vi "Swerve Drive.vi"(0 "Longitudinal - Y":dbl, 2 "Lateral - X":dbl, 3 "Rotational - Z":dbl) -> (1 "Front Left Speed":dbl, 4 "Back Left Angle":dbl, 5 "Front Left Angle":dbl, 6 "Front Right Speed":dbl, 7 "Front Right Angle":dbl, 8 "Back Left Speed":dbl, 9 "Back Right Speed":dbl, 10 "Back Right Angle":dbl)   [LabVIEW 2018]
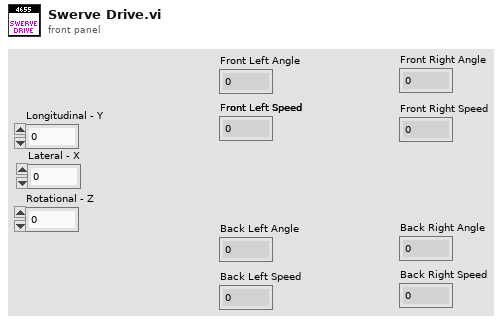
[diagram p1: front panel]
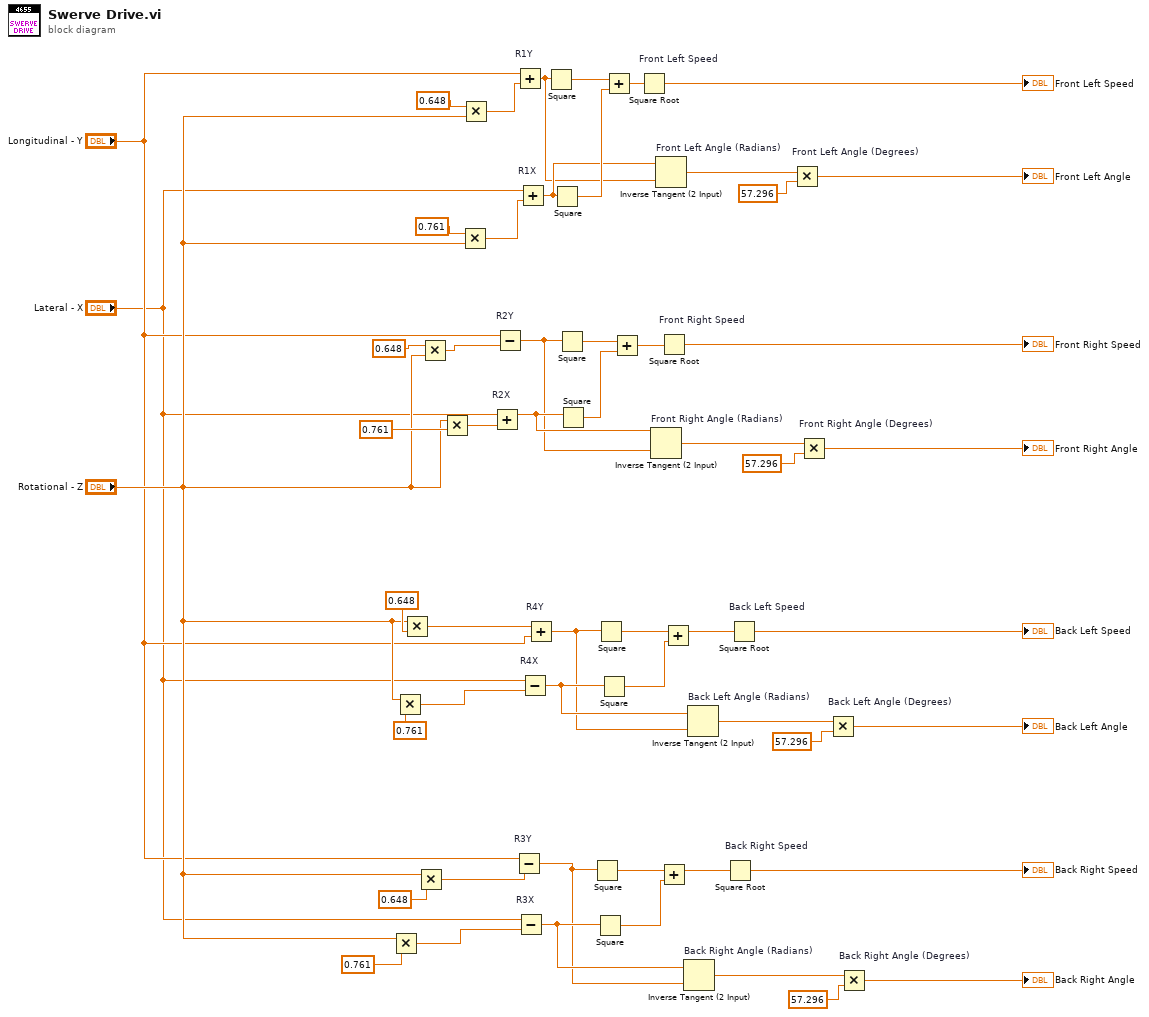
[diagram p0: block diagram]
diagram:
  n1 = Multiply(x="Rotational - Z", y=0.761 ("x")) -> (x*y=w20:dbl)
  n2 = Multiply(x="Rotational - Z", y=0.761 ("x")) -> (x*y=w30:dbl)
  n3 = Multiply(x="Rotational - Z", y=0.648 ("x")) -> (x*y=w32:dbl)
  n4 = Multiply(x="Rotational - Z", y=0.648 ("x")) -> (x*y=w11:dbl)
  n5 = Multiply(x=0.648, y="Rotational - Z") -> (x*y=w43:dbl)
  n6 = Multiply(x="Rotational - Z", y=0.761 ("x")) -> (x*y=w41:dbl)
  n7 = Multiply(x=0.761, y="Rotational - Z") -> (x*y=w52:dbl)
  n8 = Multiply(x=0.648, y="Rotational - Z") -> (x*y=w54:dbl)
  n9 = Add "R2X"(x="Lateral - X", y=w41) -> (x+y=w37:dbl)
  n10 = Subtract "R2Y"(x="Longitudinal - Y", y=w43) -> (x-y=w36:dbl)
  n11 = Subtract "R3Y"(x="Longitudinal - Y", y=w11) -> (x-y=w15:dbl)
  n12 = Add "R1Y"(x="Longitudinal - Y", y=w54) -> (x+y=w47:dbl)
  n13 = Subtract "R3X"(x="Lateral - X", y=w20) -> (x-y=w16:dbl)
  n14 = Add "R1X"(x="Lateral - X", y=w52) -> (x+y=w48:dbl)
  n15 = Subtract "R4X"(x="Lateral - X", y=w30) -> (x-y=w26:dbl)
  n16 = Add "R4Y"(x=w32, y="Longitudinal - Y") -> (x+y=w25:dbl)
  n17 = Square(x=w47) -> (x^2=w49:dbl)
  n18 = Square(x=w48) -> (x^2=w51:dbl)
  n19 = Square(x=w36) -> (x^2=w40:dbl)
  n20 = Square(x=w37) -> (x^2=w39:dbl)
  n21 = Square(x=w15) -> (x^2=w19:dbl)
  n22 = Square(x=w16) -> (x^2=w18:dbl)
  n23 = Square(x=w25) -> (x^2=w29:dbl)
  n24 = Square(x=w26) -> (x^2=w28:dbl)
  n25 = Add(x=w49, y=w51) -> (x+y=w50:dbl)
  n26 = Add(x=w40, y=w39) -> (x+y=w38:dbl)
  n27 = Square Root "Front Left Speed"(x=w50) -> (sqrt(x)=→"Front Left Speed":dbl)
  n28 = Inverse Tangent (2 Input) "Front Right Angle (Radians)"(1:w36, 2:w37) -> (0:w35:dbl)
  n29 = Inverse Tangent (2 Input) "Front Left Angle (Radians)"(1:w47, 2:w48) -> (0:w46:dbl)
  n30 = Square Root "Front Right Speed"(x=w38) -> (sqrt(x)=→"Front Right Speed":dbl)
  n31 = Add(x=w19, y=w18) -> (x+y=w17:dbl)
  n32 = Add(x=w29, y=w28) -> (x+y=w27:dbl)
  n33 = Inverse Tangent (2 Input) "Back Right Angle (Radians)"(1:w15, 2:w16) -> (0:w14:dbl)
  n34 = Inverse Tangent (2 Input) "Back Left Angle (Radians)"(1:w25, 2:w26) -> (0:w24:dbl)
  n35 = Square Root "Back Right Speed"(x=w17) -> (sqrt(x)=→"Back Right Speed":dbl)
  n36 = Square Root "Back Left Speed"(x=w27) -> (sqrt(x)=→"Back Left Speed":dbl)
  n37 = Multiply "Front Left Angle (Degrees)"(x=w46, y=57.296) -> (x*y=→"Front Left Angle":dbl)
  n38 = Multiply "Front Right Angle (Degrees)"(x=w35, y=57.296) -> (x*y=→"Front Right Angle":dbl)
  n39 = Multiply "Back Left Angle (Degrees)"(x=w24, y=57.296) -> (x*y=→"Back Left Angle":dbl)
  n40 = Multiply "Back Right Angle (Degrees)"(x=w14, y=57.296) -> (x*y=→"Back Right Angle":dbl)
